vi "Generate PWM Signal.vi"(5 "Duty Cycle Min":dbl=0.2 min=1e-06 max=0.9999 format="%.2f", 6 "Number of cycles":dbl=1.0, 7 "Duty Cycle Max":dbl=0.8 min=1e-06 max=0.9999 format="%.2f", 8 "error in":errorcluster, 9 "Number of Samples":i32=1000, 10 "Frequency":dbl=10000.0 format="%#.2f", 11 "signal type":u16(ring) items=["Sine Wave", "Triangle Wave", "Square Wave", "Sawtooth Wave"]) -> (0 "error out":errorcluster, 2 "data":cluster{"duty cycle":dbl, "frequency":dbl}[](array[cluster]))   [LabVIEW 2022 SP3]
doc: "This subVI creates an PWM waveform based on a given duty cycle min and max, number of samples and frequency."
uses:
  <vilib>/measure/NI_MABase.lvlib
panel:
  out "Waveform Graph":waveform(dbl)(graph)
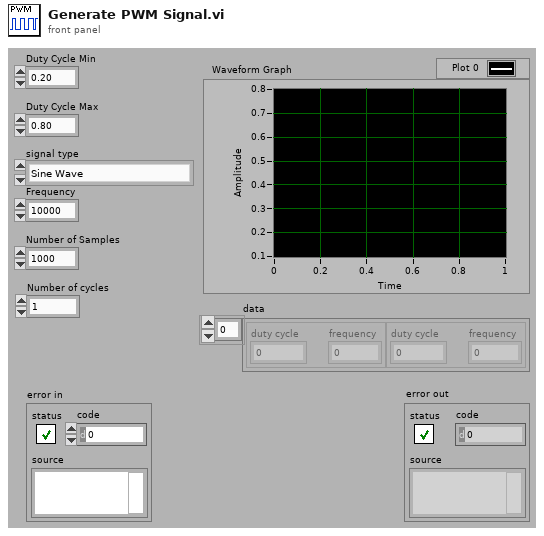
[diagram p1: front panel]
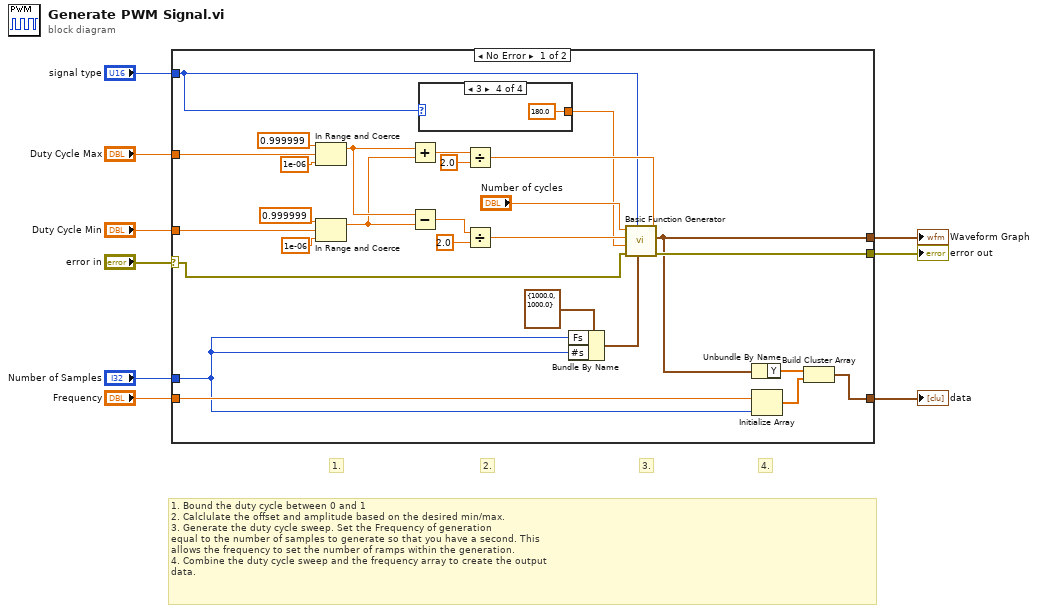
[diagram p0: block diagram]
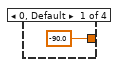
[diagram p2: hidden frame]
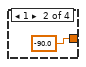
[diagram p3: hidden frame]
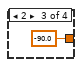
[diagram p4: hidden frame]
diagram:
  # "1. Bound the duty cycle between 0 and 1\n2. Calclulate the offset and amplitude based on the desired min/max.\n3. Generate the duty cycle sweep. Set the Frequency of generation\nequal to the number of samples to generate so that you have a second. This \nallows the frequency to set the number of ramps within the generation. \n4. Combine the duty cycle sweep and the frequency array to create the output\ndata."
  # "4."
  # "3."
  # "2."
  # "1."
  n1 = case shown="No Error" "error in" {
    selector: "error in" -> [w11 w41]
    tunnel: "Frequency" -> [w27 _]
    tunnel: [w25 _] -> w8
    tunnel: "signal type" -> [w23 _]
    tunnel: "Duty Cycle Max" -> [w21 _]
    tunnel: "Duty Cycle Min" -> [w17 _]
    tunnel: "Number of Samples" -> [w13 _]
    tunnel: [w12 w41] -> w3
    tunnel: [w10 _] -> w1
    frame No Error {
      n2 = In Range and Coerce(upper limit=0.999999, x=w21, lower limit=1e-06) -> (coerced(x)=w18:dbl)  [unwired: 1 out]
      n3 = In Range and Coerce(upper limit=0.999999, x=w17, lower limit=1e-06) -> (coerced(x)=w16:dbl)  [unwired: 1 out]
      n4 = Add(x=w18, y=w16) -> (x+y=w36:dbl)
      n5 = Subtract(x=w18, y=w16) -> (x-y=w33:dbl)
      n6 = case shown="3" w23 {
        tunnel: [-90.0 ("frequency") -90.0 ("frequency") -90.0 ("frequency") 180.0 ("frequency")] -> w22
        frame 0, Default {
        }
        frame 1 {
        }
        frame 2 {
        }
        frame 3 {
        }
      }
      n7 = Divide(x=w36, y=2.0) -> (x/y=w34:dbl)
      n8 = Divide(x=w33, y=2.0) -> (x/y=w31:dbl)
      n9 = Bundle By Name(cluster=cluster{"Fs":dbl, "#s":dbl} {"Fs"=1000.0, "#s"=1000.0} ("sampling info"), "Fs"=w13, "#s"=w13) -> (w29:cluster{"Fs":dbl, "#s":dbl})
      n10 = call <vilib>:"Basic Function Generator.vi"("offset"=w34, "sampling info"=w29, "signal type"=w23, "error in (no error)"=w11, "phase"=w22, "amplitude"=w31, "frequency"="Number of cycles") -> ("error out"=w12:errorcluster, "signal out"=w10:waveform(dbl))  [unwired: 2 in, 1 out]
      n11 = Unbundle By Name(w10) -> ("Y"=w28:dbl[])
      n12 = Initialize Array(w27, w13) -> (w26:dbl[])
      n13 = Build Cluster Array(w28, w26) -> (w25:cluster{dbl, "Frequency":dbl}[])
    }
    frame Error {
    }
  }
  "data" <- w8
  "error out" <- w3
  "Waveform Graph" <- w1
